vi "reconnect.vi"(8 "error in (no error)":errorcluster, 11 "TCPClient in":refnum<class "TCPClient.lvclass">) -> (0 "error out":errorcluster, 3 "TCPClient out":refnum<class "TCPClient.lvclass">)   [LabVIEW 2016, in "TCPClient.lvclass"]
uses:
  TCPClient.lvclass
  TCPCommunicator/TCPCommunicator.lvclass
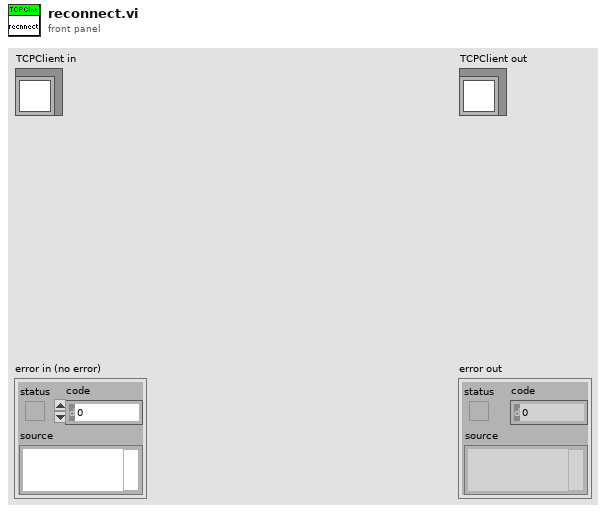
[diagram p1: front panel]
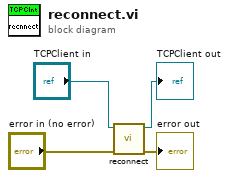
[diagram p0: block diagram]
diagram:
  n1 = call-parent "reconnect.vi"("error in (no error)"="error in (no error)", "TCPCommunicator in"="TCPClient in") -> ("error out"=→"error out":errorcluster, "TCPCommunicator out"=→"TCPClient out":refnum<class "TCPClient.lvclass">)  [unwired: 8 in]
